vi "TMC Global.vi"() -> ()   [LabVIEW 2019]
panel:
  in  "Down Readback Chan":i32=31
  in  "Up Readback Chan":i32=30
  in  "Status Chans":string="27,28,29"
  in  "Encoder Device":i32
  in  "Encoder Delay":u32=1000
  in  "Motion Delay":u32=100
  in  "Override Chan":i32=17
  in  "Down Chan":i32=16
  in  "Target Mover Device":i32=2
  in  "Up Chan":i32=15
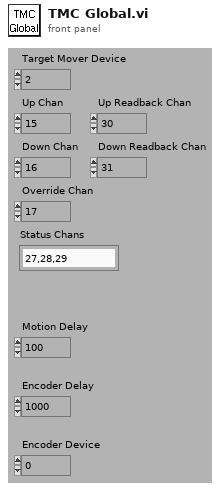
[diagram p1: front panel]
diagram:
